vi "Disconnect devices (SubVI).vi"(8 "error in (no error)":errorcluster, 9 "Force turn off MFIA":bool, 10 "Devices":T1={"MFIA"=TRUE, "Temperature controller"=TRUE, "Source meter"=TRUE}, 11 "Loop data":T2={"Persistent"={"Last file"=path "", "Last author"=""}, "Temp handle"={"Connected"=FALSE, "Temp ctrl"={"Gain (P)"=0.0, "Reset (I)"=0.0, "Rate (D)"=0, "Stabilization rate"=0.0, "Stabilization delta"=0.0, "Type"=enum."Lake Shore 325", "Custom temp ctrl"={"VISA resource name"=""}, "Lakeshore 325"={"VISA name"="", "Loop"=0, "Heater Range"=1, "Heater Resistance"=0, "Sample sensor"=0, "Fast sensor"=0, "Slow sensor"=0}}}, "Paths"={"Manual"=path "", "Settings"=path "", "Persistent"=path "", "Work dir."=path ""}, "Settings"={"MFIA"={"Address"="", "Use compensation"=FALSE, "Shut down gracefully"=FALSE}, "Temp ctrl"={"Gain (P)"=0.0, "Reset (I)"=0.0, "Rate (D)"=0, "Stabilization rate"=0.0, "Stabilization delta"=0.0, "Type"=enum."Custom", "Custom temp ctrl"={"VISA resource name"=""}, "Lakeshore 325"={"VISA name"="", "Loop"=0, "Heater Range"=0, "Heater Resistance"=0, "Sample sensor"=0, "Fast sensor"=0, "Slow sensor"=0}}, "Source-meter"={"Type"=enum."Custom", "Custom source-meter"={"VISA resource name"=""}, "Keithley 2600"={"VISA name"=""}}, "Other"={"Enable OriginLab"=FALSE, "Reader mode"=FALSE}, "Defaults"={"IV properties"={"T"=0.0, "Vstart"=-0.5, "Vstop"=0.5, "Vpoints"=10.0, "Settling"=0.01, "I limit"=0.1, "Log mapping"=FALSE, "Averaging"=0.0}, "CV properties"={"T"=0.0, "Vstart"=-0.5, "Vstop"=0.5, "Vpoints"=10.0, "Precision"=enum."Normal", "Test signal"=0.01, "Auto I range"=FALSE, "Test frequency"=100000.0, "I range"=-2.0, "V range"=10.0, "Log mapping"=FALSE, "Rel perm"=0.0, "Area"=0.0}, "DLTS properties"={"Tstart"=0.0, "Instant start"=FALSE, "Tstop"=0.0, "T rate"=0.0, "Test signal"=0.0, "Test frequency"=0.0, "Bandwidth"=0.0, "Averaging"=0.0, "Vbias"=0.0, "Vpulse"=0.0, "pulse length"=0.0, "Pulse 2"=FALSE, "Vpulse 2"=0.0, "pulse length 2"=0.0, "I range"=-2.0, "V range"=10.0, "Emission rate"=[], "Sampling rate"=0.0, "Acq. delay"=0.0}, "LDLTS properties"={"T"=0.0, "Test signal"=0.0, "Test frequency"=0.0, "Bandwidth"=0.0, "Averaging"=0.0, "Vbias"=0.0, "Vpulse"=0.0, "pulse length"=0.0, "Pulse 2"=FALSE, "Vpulse 2"=0.0, "pulse length 2"=0.0, "I range"=-2.0, "V range"=10.0, "Sampling rate"=0.0, "Acq. delay"=0.0, "Sampling time"=0.0}}}, "Software version"=0.0, "MFIA handle"={"ziHandle"={"handleValid"=FALSE, "Conn"=0, "Path Prefix"="", "Handle"=0, "Connected"=FALSE, "Clockbase(s)"=0.0}, "Selected device"="", "ziModHandle"={"handleValid"=FALSE, "Conn"=0, "ModHandle"=0, "moduleID"="", "Path Prefix"=""}}, "Source-meter handle"={"Connected"=FALSE, "Source-meter"={"Type"=enum."Custom", "Custom source-meter"={"VISA resource name"=""}, "Keithley 2600"={"VISA name"=""}}}} {"MFIA handle"."ziModHandle"."ModHandle" format="0x%08x"; "MFIA handle"."ziModHandle"."Conn" format="0x%08x"; "MFIA handle"."ziHandle"."Handle" format="0x%08x"; "MFIA handle"."ziHandle"."Conn" format="0x%08x"; "Settings"."Defaults"."LDLTS properties"."V range" items=["10mV"=0.01, "100mV"=0.1, "1V"=1.0, "10V"=10.0]; "Settings"."Defaults"."LDLTS properties"."I range" items=["100nA"=-7.0, "1µA"=-6.0, "10µA"=-5.0, "100µA"=-4.0, "1mA"=-3.0, "10mA"=-2.0]; "Settings"."Defaults"."DLTS properties"."V range" items=["10mV"=0.01, "100mV"=0.1, "1V"=1.0, "10V"=10.0]; "Settings"."Defaults"."DLTS properties"."I range" items=["10mV"=0.01, "100mV"=0.1, "1V"=1.0, "10V"=10.0]; "Settings"."Defaults"."CV properties"."V range" items=["10mV"=0.01, "100mV"=0.1, "1V"=1.0, "10V"=10.0]; "Settings"."Defaults"."CV properties"."I range" items=["100nA"=-7.0, "1µA"=-6.0, "10µA"=-5.0, "100µA"=-4.0, "1mA"=-3.0, "10mA"=-2.0]; "Settings"."Defaults"."IV properties"."Settling" min=0.0 max=65535.0; "Settings"."Temp ctrl"."Lakeshore 325"."Slow sensor" items=["A", "B"]; "Settings"."Temp ctrl"."Lakeshore 325"."Fast sensor" items=["A", "B"]; "Settings"."Temp ctrl"."Lakeshore 325"."Sample sensor" items=["A", "B"]; "Settings"."Temp ctrl"."Lakeshore 325"."Heater Resistance" items=["25 Ohm"=1, "50 Ohm"=2]; "Settings"."Temp ctrl"."Lakeshore 325"."Heater Range" items=["Off", "Low (loop 1) or On (loop 2)", "High (loop 1)"]; "Settings"."Temp ctrl"."Lakeshore 325"."Loop" items=["Loop 1"=1, "Loop 2"=2]; "Temp handle"."Temp ctrl"."Lakeshore 325"."Slow sensor" items=["A", "B"]; "Temp handle"."Temp ctrl"."Lakeshore 325"."Fast sensor" items=["A", "B"]; "Temp handle"."Temp ctrl"."Lakeshore 325"."Sample sensor" items=["A", "B"]; "Temp handle"."Temp ctrl"."Lakeshore 325"."Heater Resistance" items=["25 Ohm"=1, "50 Ohm"=2]; "Temp handle"."Temp ctrl"."Lakeshore 325"."Heater Range" items=["Off", "Low (loop 1) or On (loop 2)", "High (loop 1)"]; "Temp handle"."Temp ctrl"."Lakeshore 325"."Loop" items=["Loop 1"=1, "Loop 2"=2]}) -> (0 "Error Out":errorcluster, 3 "Loop data out":T2={"Persistent"={"Last file"=path "", "Last author"=""}, "Temp handle"={"Connected"=FALSE, "Temp ctrl"={"Gain (P)"=0.0, "Reset (I)"=0.0, "Rate (D)"=0, "Stabilization rate"=0.0, "Stabilization delta"=0.0, "Type"=enum."Lake Shore 325", "Custom temp ctrl"={"VISA resource name"=""}, "Lakeshore 325"={"VISA name"="", "Loop"=0, "Heater Range"=1, "Heater Resistance"=0, "Sample sensor"=0, "Fast sensor"=0, "Slow sensor"=0}}}, "Paths"={"Manual"=path "", "Settings"=path "", "Persistent"=path "", "Work dir."=path ""}, "Settings"={"MFIA"={"Address"="", "Use compensation"=TRUE, "Shut down gracefully"=FALSE}, "Temp ctrl"={"Gain (P)"=0.0, "Reset (I)"=0.0, "Rate (D)"=0, "Stabilization rate"=0.0, "Stabilization delta"=0.0, "Type"=enum."Lake Shore 325", "Custom temp ctrl"={"VISA resource name"=""}, "Lakeshore 325"={"VISA name"="", "Loop"=0, "Heater Range"=1, "Heater Resistance"=0, "Sample sensor"=0, "Fast sensor"=0, "Slow sensor"=0}}, "Source-meter"={"Type"=enum."Custom", "Custom source-meter"={"VISA resource name"=""}, "Keithley 2600"={"VISA name"=""}}, "Other"={"Enable OriginLab"=FALSE, "Reader mode"=FALSE}, "Defaults"={"IV properties"={"T"=0.0, "Vstart"=-0.5, "Vstop"=0.5, "Vpoints"=10.0, "Settling"=0.01, "I limit"=0.1, "Log mapping"=FALSE, "Averaging"=0.0}, "CV properties"={"T"=0.0, "Vstart"=-0.5, "Vstop"=0.5, "Vpoints"=10.0, "Precision"=enum."Normal", "Test signal"=0.01, "Auto I range"=FALSE, "Test frequency"=100000.0, "I range"=-2.0, "V range"=10.0, "Log mapping"=FALSE, "Rel perm"=0.0, "Area"=0.0}, "DLTS properties"={"Tstart"=0.0, "Instant start"=FALSE, "Tstop"=0.0, "T rate"=0.0, "Test signal"=0.0, "Test frequency"=0.0, "Bandwidth"=0.0, "Averaging"=0.0, "Vbias"=0.0, "Vpulse"=0.0, "pulse length"=0.0, "Pulse 2"=FALSE, "Vpulse 2"=0.0, "pulse length 2"=0.0, "I range"=-2.0, "V range"=10.0, "Emission rate"=[], "Sampling rate"=0.0, "Acq. delay"=0.0}, "LDLTS properties"={"T"=0.0, "Test signal"=0.0, "Test frequency"=0.0, "Bandwidth"=0.0, "Averaging"=0.0, "Vbias"=0.0, "Vpulse"=0.0, "pulse length"=0.0, "Pulse 2"=FALSE, "Vpulse 2"=0.0, "pulse length 2"=0.0, "I range"=-2.0, "V range"=10.0, "Sampling rate"=0.0, "Acq. delay"=0.0, "Sampling time"=0.0}}}, "Software version"=0.0, "MFIA handle"={"ziHandle"={"handleValid"=FALSE, "Conn"=0, "Path Prefix"="", "Handle"=0, "Connected"=FALSE, "Clockbase(s)"=0.0}, "Selected device"="", "ziModHandle"={"handleValid"=FALSE, "Conn"=0, "ModHandle"=0, "moduleID"="", "Path Prefix"=""}}, "Source-meter handle"={"Connected"=FALSE, "Source-meter"={"Type"=enum."Custom", "Custom source-meter"={"VISA resource name"=""}, "Keithley 2600"={"VISA name"=""}}}} {"MFIA handle"."ziModHandle"."ModHandle" format="0x%08x"; "MFIA handle"."ziModHandle"."Conn" format="0x%08x"; "MFIA handle"."ziHandle"."Handle" format="0x%08x"; "MFIA handle"."ziHandle"."Conn" format="0x%08x"; "Settings"."Defaults"."LDLTS properties"."V range" items=["10mV"=0.01, "100mV"=0.1, "1V"=1.0, "10V"=10.0]; "Settings"."Defaults"."LDLTS properties"."I range" items=["100nA"=-7.0, "1µA"=-6.0, "10µA"=-5.0, "100µA"=-4.0, "1mA"=-3.0, "10mA"=-2.0]; "Settings"."Defaults"."DLTS properties"."V range" items=["10mV"=0.01, "100mV"=0.1, "1V"=1.0, "10V"=10.0]; "Settings"."Defaults"."DLTS properties"."I range" items=["10mV"=0.01, "100mV"=0.1, "1V"=1.0, "10V"=10.0]; "Settings"."Defaults"."CV properties"."V range" items=["10mV"=0.01, "100mV"=0.1, "1V"=1.0, "10V"=10.0]; "Settings"."Defaults"."CV properties"."I range" items=["100nA"=-7.0, "1µA"=-6.0, "10µA"=-5.0, "100µA"=-4.0, "1mA"=-3.0, "10mA"=-2.0]; "Settings"."Defaults"."IV properties"."Settling" min=0.0 max=65535.0; "Settings"."Temp ctrl"."Lakeshore 325"."Slow sensor" items=["A", "B"]; "Settings"."Temp ctrl"."Lakeshore 325"."Fast sensor" items=["A", "B"]; "Settings"."Temp ctrl"."Lakeshore 325"."Sample sensor" items=["A", "B"]; "Settings"."Temp ctrl"."Lakeshore 325"."Heater Resistance" items=["25 Ohm"=1, "50 Ohm"=2]; "Settings"."Temp ctrl"."Lakeshore 325"."Heater Range" items=["Off", "Low (loop 1) or On (loop 2)", "High (loop 1)"]; "Settings"."Temp ctrl"."Lakeshore 325"."Loop" items=["Loop 1"=1, "Loop 2"=2]; "Temp handle"."Temp ctrl"."Lakeshore 325"."Slow sensor" items=["A", "B"]; "Temp handle"."Temp ctrl"."Lakeshore 325"."Fast sensor" items=["A", "B"]; "Temp handle"."Temp ctrl"."Lakeshore 325"."Sample sensor" items=["A", "B"]; "Temp handle"."Temp ctrl"."Lakeshore 325"."Heater Resistance" items=["25 Ohm"=1, "50 Ohm"=2]; "Temp handle"."Temp ctrl"."Lakeshore 325"."Heater Range" items=["Off", "Low (loop 1) or On (loop 2)", "High (loop 1)"]; "Temp handle"."Temp ctrl"."Lakeshore 325"."Loop" items=["Loop 1"=1, "Loop 2"=2]})   [LabVIEW 2019]
doc: "Terminates connection with hardware, displays dialog"
uses:
  Type defs/Loop data Type Def.ctl
  Type defs/Persistent Type Def.ctl
  Type defs/Temp handle Type Def.ctl
  Type defs/Temp ctrl Type Def.ctl
  Custom devices/Custom temp ctrl settings.ctl
  Type defs/Paths Type Def.ctl
  Type defs/Settings Type Def.ctl
  Type defs/Imps Type Def.ctl
  Type defs/Source-meter Type Def.ctl
  Custom devices/Custom source-meter settings.ctl
  Type defs/Other settings Type Def.ctl
  Type defs/IV properties Type Def.ctl
  Type defs/CV properties Type Def.ctl
  Type defs/DLTS properties Type Def.ctl
  Type defs/LDLTS properties Type Def.ctl
  Type defs/MFIA handle Type Def.ctl
  <instrlib>/Zurich Instruments LabOne/Public/ziTypeHandle.ctl
  <instrlib>/Zurich Instruments LabOne/Public/Modules/ziTypeModHandle.ctl
  Type defs/Source-meter handle Type Def.ctl
  <instrlib>/Zurich Instruments LabOne/Public/Configure/ziSetValueDouble.vi
  <instrlib>/Zurich Instruments LabOne/Zurich Instruments LabOne.lvlib
panel:
  out "Animated picture":u16(ring)
  out "String":string
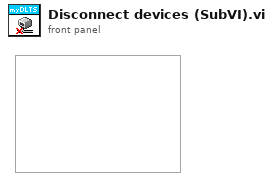
[diagram p1: front panel]
types:
  T1 = cluster{"MFIA":bool, "Temperature controller":bool, "Source meter":bool}
  T2 = typedef "Loop data Type Def.ctl" = cluster{"Persistent":T3, "Temp handle":T4, "Paths":T7, "Settings":T8, "Software version":dbl, "MFIA handle":T17, "Source-meter handle":T20}
  T3 = typedef "Persistent Type Def.ctl" = cluster{"Last file":path, "Last author":string}
  T4 = typedef "Temp handle Type Def.ctl" = cluster{"Connected":bool, "Temp ctrl":T5}
  T5 = typedef "Temp ctrl Type Def.ctl" = cluster{"Gain (P)":dbl, "Reset (I)":dbl, "Rate (D)":u16, "Stabilization rate":dbl, "Stabilization delta":dbl, "Type":enum16{"Custom", "Lake Shore 325"}, "Custom temp ctrl":T6, "Lakeshore 325":cluster{"VISA name":refnum<visa-resource-name>, "Loop":u16, "Heater Range":u16, "Heater Resistance":u16, "Sample sensor":u16, "Fast sensor":u16, "Slow sensor":u16}}
  T6 = typedef "Custom temp ctrl settings.ctl" = cluster{"VISA resource name":refnum<visa-resource-name>}
  T7 = typedef "Paths Type Def.ctl" = cluster{"Manual":path, "Settings":path, "Persistent":path, "Work dir.":path}
  T8 = typedef "Settings Type Def.ctl" = cluster{"MFIA":T9, "Temp ctrl":T5, "Source-meter":T10, "Other":T12, "Defaults":cluster{"IV properties":T13, "CV properties":T14, "DLTS properties":T15, "LDLTS properties":T16}}
  T9 = typedef "Imps Type Def.ctl" = cluster{"Address":string, "Use compensation":bool, "Shut down gracefully":bool}
  T10 = typedef "Source-meter Type Def.ctl" = cluster{"Type":enum16{"Custom", "Keithley 2600"}, "Custom source-meter":T11, "Keithley 2600":cluster{"VISA name":refnum<visa-resource-name>}}
  T11 = typedef "Custom source-meter settings.ctl" = cluster{"VISA resource name":refnum<visa-resource-name>}
  T12 = typedef "Other settings Type Def.ctl" = cluster{"Enable OriginLab":bool, "Reader mode":bool}
  T13 = typedef "IV properties Type Def.ctl" = cluster{"T":dbl[unit], "Vstart":dbl[unit], "Vstop":dbl[unit], "Vpoints":dbl, "Settling":dbl[unit], "I limit":dbl[unit], "Log mapping":bool, "Averaging":dbl}
  T14 = typedef "CV properties Type Def.ctl" = cluster{"T":dbl[unit], "Vstart":dbl[unit], "Vstop":dbl[unit], "Vpoints":dbl, "Precision":enum16{"Low (Fast)", "Normal", "High (Slow)"}, "Test signal":dbl[unit], "Auto I range":bool, "Test frequency":dbl[unit], "I range":dbl, "V range":dbl[unit], "Log mapping":bool, "Rel perm":dbl, "Area":dbl[unit]}
  T15 = typedef "DLTS properties Type Def.ctl" = cluster{"Tstart":dbl[unit], "Instant start":bool, "Tstop":dbl[unit], "T rate":dbl[unit], "Test signal":dbl[unit], "Test frequency":dbl[unit], "Bandwidth":dbl[unit], "Averaging":dbl, "Vbias":dbl[unit], "Vpulse":dbl[unit], "pulse length":dbl[unit], "Pulse 2":bool, "Vpulse 2":dbl[unit], "pulse length 2":dbl[unit], "I range":dbl, "V range":dbl[unit], "Emission rate":dbl[unit][], "Sampling rate":dbl[unit], "Acq. delay":dbl[unit]}
  T16 = typedef "LDLTS properties Type Def.ctl" = cluster{"T":dbl[unit], "Test signal":dbl[unit], "Test frequency":dbl[unit], "Bandwidth":dbl[unit], "Averaging":dbl, "Vbias":dbl[unit], "Vpulse":dbl[unit], "pulse length":dbl[unit], "Pulse 2":bool, "Vpulse 2":dbl[unit], "pulse length 2":dbl[unit], "I range":dbl, "V range":dbl[unit], "Sampling rate":dbl[unit], "Acq. delay":dbl[unit], "Sampling time":dbl[unit]}
  T17 = typedef "MFIA handle Type Def.ctl" = cluster{"ziHandle":T18, "Selected device":string, "ziModHandle":T19}
  T18 = typedef "Zurich Instruments LabOne.lvlib/ziTypeHandle.ctl" = cluster{"handleValid":bool, "Conn":u64, "Path Prefix":string, "Handle":u64, "Connected":bool, "Clockbase(s)":dbl}
  T19 = typedef "Zurich Instruments LabOne.lvlib/ziTypeModHandle.ctl" = cluster{"handleValid":bool, "Conn":u64, "ModHandle":u64, "moduleID":string, "Path Prefix":string}
  T20 = typedef "Source-meter handle Type Def.ctl" = cluster{"Connected":bool, "Source-meter":T10}
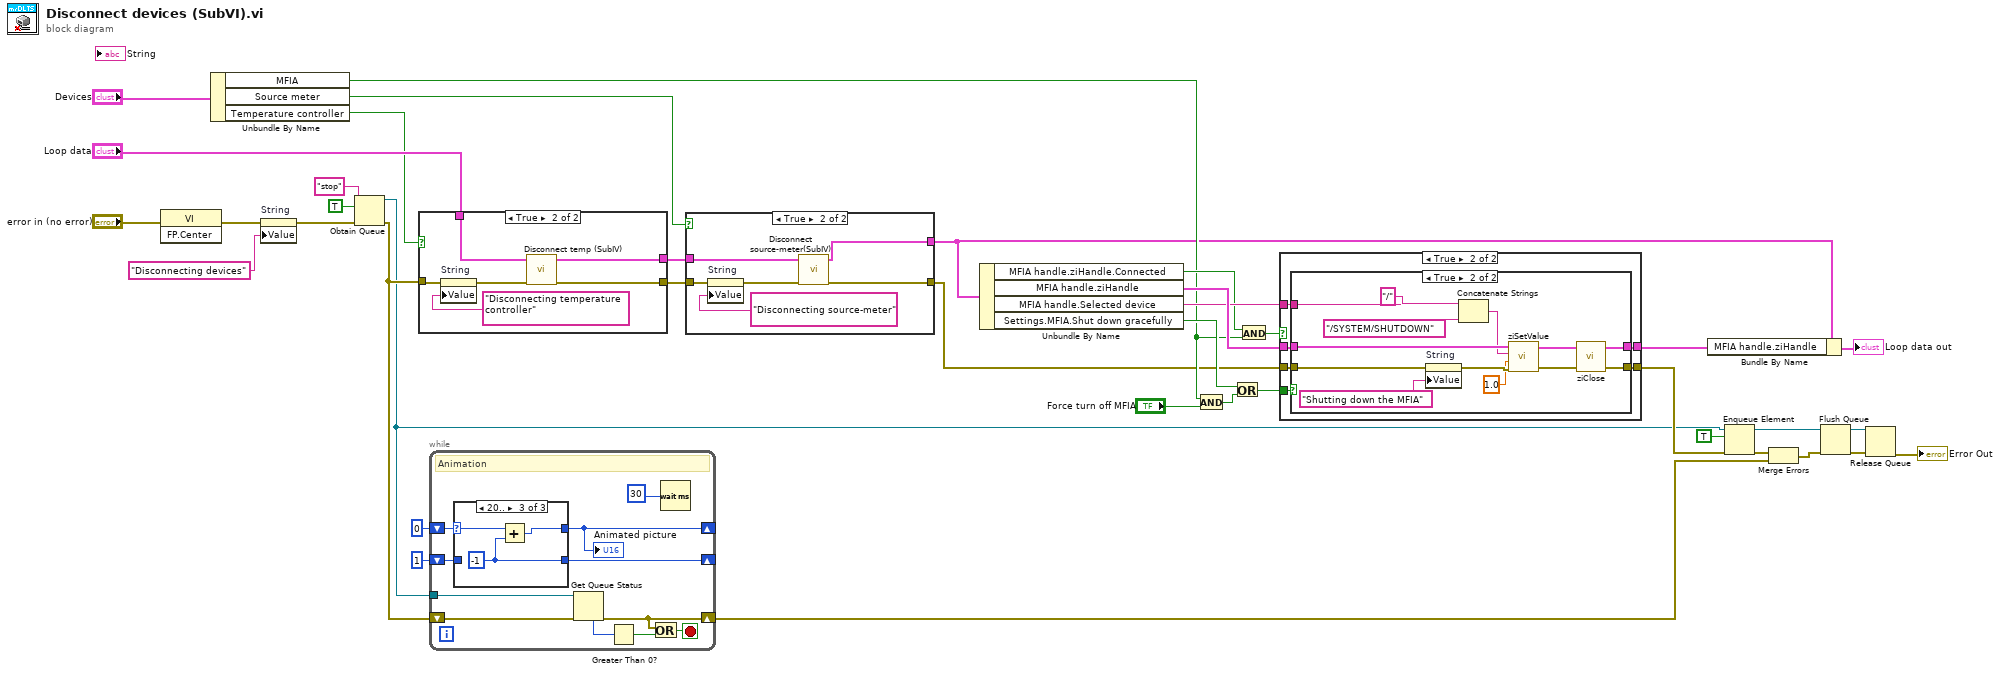
[diagram p0: block diagram]
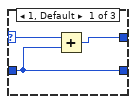
[diagram p2: hidden frame]
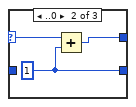
[diagram p3: hidden frame]
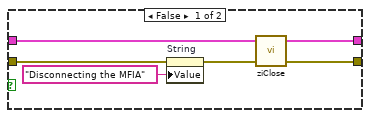
[diagram p6: hidden frame]
diagram:
  n1 = invoke class="VI" method="FP.Center"(error in="error in (no error)") -> (error out=w21:errorcluster)  [unwired: 2 in, 2 out]
  n2 = Unbundle By Name("Devices") -> ("MFIA"=w11:bool, "Source meter"=w6:bool, "Temperature controller"=w13:bool)
  n3 = property on="String" class="Str"(error in=w21, "Value"="Disconnecting devices" ("String")) -> (error out=w24:errorcluster)  [unwired: 1 in, 1 out]
  n4 = Obtain Queue(name (unnamed)="stop", element data type=TRUE, error in (no error)=w24) -> (queue out=w2:refnum<queue>, error out=w3:errorcluster)  [unwired: 2 in, 1 out]
  n5 = case shown="True" w13 {
    tunnel: w3 -> [w39 w45]
    tunnel: "Loop data" -> [w40 w41]
    tunnel: [w40 w42] -> w10
    tunnel: [w39 w43] -> w7
    frame False {
    }
    frame True {
      n6 = property on="String" class="Str"(error in=w45, "Value"="Disconnecting temperature controller" ("String")) -> (error out=w44:errorcluster)  [unwired: 1 in, 1 out]
      n7 = call "Disconnect temp (SubIV).vi"("Error In"=w44, "Loop data In"=w41) -> ("Error Out"=w43:errorcluster, "Loop data Out"=w42:T2)  [unwired: 8 in]
    }
  }
  n8 = while {
    shift-right: [w56] -> _
    shift-left: u16 0 -> [w57]
    shift-right: [w53] -> _
    shift-left: i16 1 ("y") -> [w54]
    shift-right: [w49] -> w1
    shift-left: w3 -> [w48]
    tunnel: w2 -> [w47]
    stop <- w50 stop-if-true
    # "Animation"
    n9 = case shown="20.." w57 {
      selector: w57 -> [w60 w63 w66]
      tunnel: [w59 w62 w65] -> w56
      tunnel: w54 -> [w58 _ _]
      tunnel: [w58 w61 w64] -> w53
      frame 1, Default {
        n10 = Add(x=w60, y=w58) -> (x+y=w59:u16)
      }
      frame ..0 {
        w61 = i16 1 ("y")
        n11 = Add(x=w63, y=w61) -> (x+y=w62:u16)
      }
      frame 20.. {
        w64 = i16 -1 ("y")
        n12 = Add(x=w66, y=w64) -> (x+y=w65:u16)
      }
    }
    "Animated picture" <- w56
    n13 = Get Queue Status(queue=w47, error in (no error)=w48) -> (error out=w49:errorcluster, # elements in queue=w52:i32)  [unwired: 1 in, 6 out]
    n14 = Greater Than 0?(x=w52) -> (x > 0?=w51:bool)
    n15 = Or(x=w49, y=w51) -> (x .or. y?=w50:bool)
    n16 = Wait (ms)(milliseconds to wait=u32 30) -> ()  [unwired: 1 out]
  }
  n17 = case shown="True" w6 {
    tunnel: w7 -> [w67 w73]
    tunnel: w10 -> [w68 w72]
    tunnel: [w68 w69] -> w8
    tunnel: [w67 w70] -> w9
    frame False {
    }
    frame True {
      n18 = property on="String" class="Str"(error in=w73, "Value"="Disconnecting source-meter" ("String")) -> (error out=w71:errorcluster)  [unwired: 1 in, 1 out]
      n19 = call "Disconnect source-meter(SubIV).vi"("Error In"=w71, "Loop data In"=w72) -> ("Error Out"=w70:errorcluster, "Loop data Out"=w69:T2)  [unwired: 8 in]
    }
  }
  n20 = Unbundle By Name(w8) -> ("MFIA handle.ziHandle.Connected"=w12:bool, "MFIA handle.ziHandle"=w37:T18, "MFIA handle.Selected device"=w19:string, "Settings.MFIA.Shut down gracefully"=w20:bool)
  n21 = And(x=w11, y="Force turn off MFIA") -> (x .and. y?=w14:bool)
  n22 = Or(x=w20, y=w14) -> (x .or. y?=w16:bool)
  n23 = And(x=w12, y=w11) -> (x .and. y?=w17:bool)
  n24 = case shown="True" w17 {
    tunnel: w37 -> [w76 w82]
    tunnel: w9 -> [w75 w81]
    tunnel: [w75 w79] -> w30
    tunnel: [w76 w80] -> w36
    tunnel: w16 -> [_ w78]
    tunnel: w19 -> [_ w77]
    frame False {
    }
    frame True {
      n25 = case shown="True" w78 {
        tunnel: w82 -> [w88 w94]
        tunnel: w81 -> [w85 w99]
        tunnel: [w87 w101] -> w80
        tunnel: [w83 w98] -> w79
        tunnel: w77 -> [_ w90]
        frame False {
          n26 = property on="String" class="Str"(error in=w85, "Value"="Disconnecting the MFIA" ("String")) -> (error out=w84:errorcluster)  [unwired: 1 in, 1 out]
          n27 = call <instrlib>:"ziClose.vi"("Error In"=w84, "Handle In"=w88) -> ("Error Out"=w83:errorcluster, "Handle Out"=w87:T18)  [unwired: 2 in]
        }
        frame True {
          n28 = property on="String" class="Str"(error in=w99, "Value"="Shutting down the MFIA" ("String")) -> (error out=w97:errorcluster)  [unwired: 1 in, 1 out]
          n29 = Concatenate Strings("/" ("Path"), w90, "/SYSTEM/SHUTDOWN" ("string")) -> (w92:string)
          n30 = call-poly <instrlib>:"ziSetValue.vi"("Error In"=w97, "Value"=1.0, "Path"=w92, "Handle In"=w94) -> ("Error Out"=w96:errorcluster, "Handle Out"=w95:T18)  [unwired: 1 in]
          n31 = call <instrlib>:"ziClose.vi"("Error In"=w96, "Handle In"=w95) -> ("Error Out"=w98:errorcluster, "Handle Out"=w101:T18)  [unwired: 2 in]
        }
      }
    }
  }
  n32 = Bundle By Name(cluster=w8, "MFIA handle.ziHandle"=w36) -> (→"Loop data out":T2)
  n33 = Enqueue Element(queue=w2, element=TRUE ("notification"), error in (no error)=w30) -> (queue out=w27:refnum<queue>, error out=w29:errorcluster)  [unwired: 1 in, 1 out]
  n34 = Merge Errors(w29, w1) -> (w25:errorcluster)
  n35 = Flush Queue(queue=w27, error in (no error)=w25) -> (queue out=w34:refnum<queue>, error out=w33:errorcluster)  [unwired: 1 out]
  n36 = Release Queue(queue=w34, error in (no error)=w33) -> (error out=→"Error Out":errorcluster)  [unwired: 1 in, 2 out]
